vi "Duplicate.vi"(8 "error in":errorcluster, 10 "parameters":variant, 11 "DIO Channel in":refnum<class "Digital IO Channel.lvclass">) -> (0 "error out":errorcluster, 3 "DIO Channel copy":refnum<class "Digital IO Channel.lvclass">)   [LabVIEW 2025, in "Digital IO.lvlib" / "Digital IO Channel.lvclass"]
doc: "Implements the specific behavior of a node when it is being duplicated\nCan be used to change the name of the new node for example adding Copy to it. \nCopyright 2017 National Instruments Corporation\n\nLicensed under the Apache License, Version 2.0 (the \"License\"); you may not use this file except in compliance with the License. You may obtain a copy of the License at http://www.apache.org/licenses/LICENSE-2.0\nUnless required by applicable law or agreed to in writing, software distributed under the License is distributed on an \"AS IS\" BASIS, WITHOUT WARRANTIES OR CONDITIONS OF ANY KIND, either express or implied. See the License for the specific language governing permissions and limitations under the License."
uses:
  Digital IO Channel.lvclass
  Digital IO Channel.lvclass/Digital IO Channel.ctl
  Digital IO Channel configuration/Digital IO Channel configuration.lvclass
  Users/Public/Documents/Sandia National Labs/TSS Plugin/Abstract Engine.lvlibp/Plugin/Abstract/Abstract Channel/Abstract Channel.lvclass
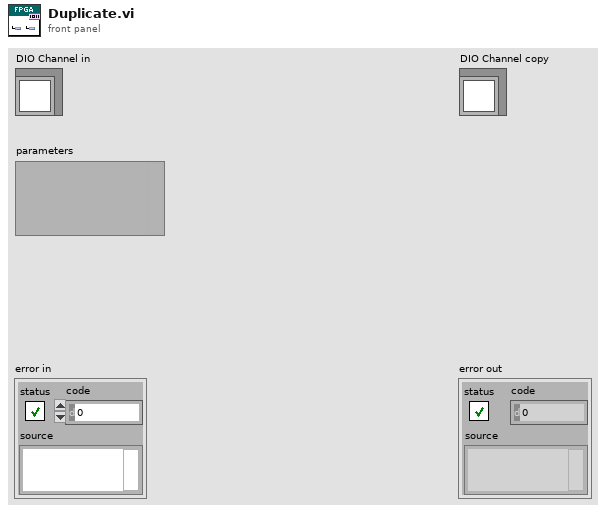
[diagram p1: front panel]
types:
  T1 = cluster{"Address":string, "SW Alias":string, "Enabled":bool, "Type":string, "Description":string}
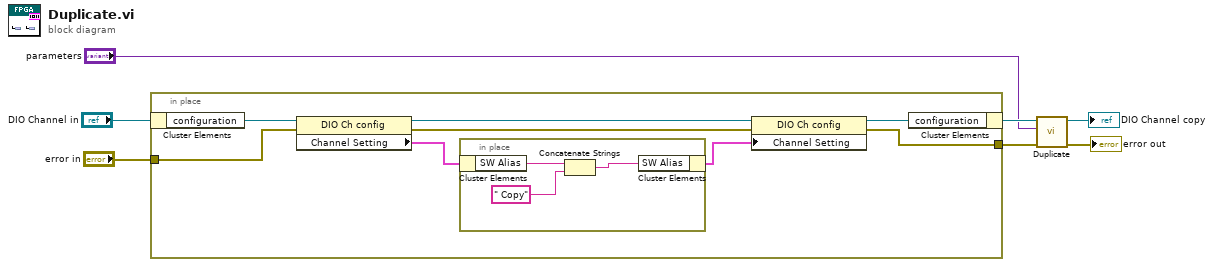
[diagram p0: block diagram]
diagram:
  n1 = in-place {
    in-place-border: "error in" -> [w11]
    in-place-border: [w9] -> w2
    n2 = in-place-cluster #1("DIO Channel in") -> ("configuration"=w15:refnum<class "Digital IO Channel configuration.lvclass">)
    n3 = property class="DIO Ch config"(reference=w15, error in=w11) -> (reference out=w13:refnum<class "Digital IO Channel configuration.lvclass">, error out=w10:errorcluster, "Channel Setting"=w12:T1)
    n4 = in-place {
      n5 = in-place-cluster #2(w12) -> ("SW Alias"=w18:string)
      n6 = Concatenate Strings(w18, " Copy") -> (w17:string)
      n7 = in-place-cluster #2("SW Alias"=w17) -> (w8:T1)
    }
    n8 = property class="DIO Ch config"(reference=w13, error in=w10, "Channel Setting"=w8) -> (reference out=w14:refnum<class "Digital IO Channel configuration.lvclass">, error out=w9:errorcluster)
    n9 = in-place-cluster #1("configuration"=w14) -> (w7:refnum<class "Digital IO Channel.lvclass">)
  }
  n10 = call-parent "Duplicate.vi"("error in"=w2, "parameters"="parameters", "CEF_Serialize node in"=w7) -> ("error out"=→"error out":errorcluster, "CEF_Serialize node out"=→"DIO Channel copy":refnum<class "Digital IO Channel.lvclass">)  [unwired: 7 in]
